vi "Set 2D Picture Ring.vi"(8 "error in (no error)":errorcluster, 10 "Selection Grid":T1) -> (0 "error out":errorcluster, 1 "Valid":bool, 3 "Grassfire out":refnum<class "Grassfire.lvclass">)   [LabVIEW 2019, in "Grassfire.lvclass"]
uses:
  Grassfire.lvclass
  Shared/Selection--array.ctl
  Shared/Selection--picture ring.ctl
  Grassfire.lvclass/Grassfire.ctl
  Node/Node.lvclass
  Address/Address.lvclass
  Shared/Shared.lvlib
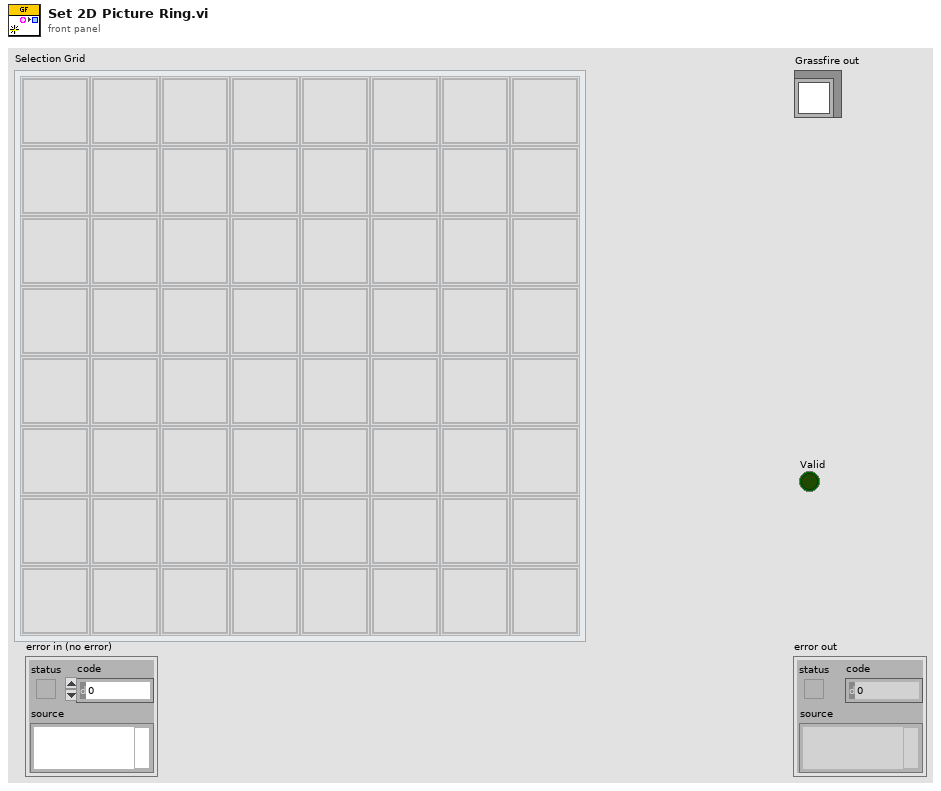
[diagram p1: front panel]
types:
  T1 = typedef "Shared.lvlib/Selection--array.ctl" = cluster{"Grid Value":T2}[][]
  T2 = typedef "Shared.lvlib/Selection--picture ring.ctl" = i64
  T3 = cluster{"Empty":refnum<class "Node.lvclass">, "Blocked":refnum<class "Node.lvclass">, "Start":refnum<class "Node.lvclass">, "End":refnum<class "Node.lvclass">, "Path":refnum<class "Node.lvclass">}
  T4 = map{refnum<class "Address.lvclass">, refnum<class "Node.lvclass">}
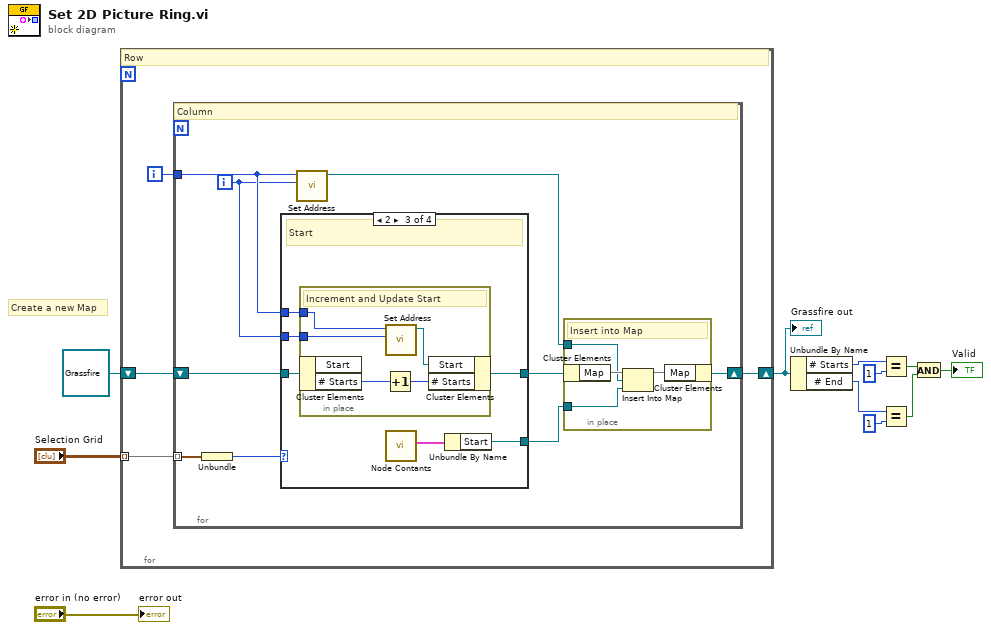
[diagram p0: block diagram]
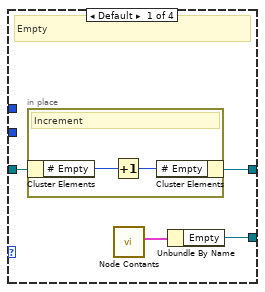
[diagram p2: hidden frame]
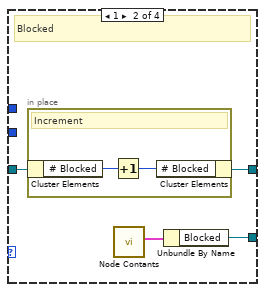
[diagram p3: hidden frame]
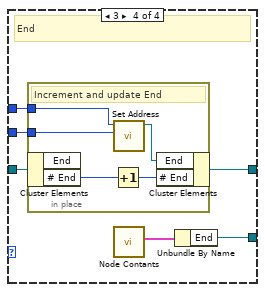
[diagram p4: hidden frame]
diagram:
  # "Create a new Map"
  n1 = for {
    tunnel: "Selection Grid" -> [w15] mode=indexing
    shift-right: [w12] -> w1
    shift-left: refnum<class "Grassfire.lvclass"> refnum ("Grassfire out") -> [w13]
    i -> [w14]
    # "Row"
    n2 = for {
      tunnel: w15 -> [w24] mode=indexing
      tunnel: w14 -> [w23]
      shift-right: [w18] -> w12
      shift-left: w13 -> [w20]
      i -> [w22]
      # "Column"
      n3 = Unbundle(w24) -> ("Grid Value"=w21:T2)
      n4 = case shown="2" w21 {
        tunnel: w20 -> [w32 w38 w46 w57]
        tunnel: [w31 w37 w45 w56] -> w19
        tunnel: w23 -> [_ _ w44 w55]
        tunnel: w22 -> [_ _ w43 w54]
        tunnel: [w29 w35 w41 w52] -> w16
        frame Default {
          # "Empty"
          n5 = in-place {
            # "Increment"
            n6 = in-place-cluster #1(w32) -> ("# Empty"=w34:i32)
            n7 = Increment(x=w34) -> (x+1=w33:i32)
            n8 = in-place-cluster #1("# Empty"=w33) -> (w31:refnum<class "Grassfire.lvclass">)
          }
          n9 = call "Node Contants.vi"() -> ("Constants"=w30:T3)  [unwired: 10 in, 1 out]
          n10 = Unbundle By Name(w30) -> ("Empty"=w29:refnum<class "Node.lvclass">)
        }
        frame 1 {
          # "Blocked"
          n11 = in-place {
            # "Increment"
            n12 = in-place-cluster #2(w38) -> ("# Blocked"=w40:i32)
            n13 = Increment(x=w40) -> (x+1=w39:i32)
            n14 = in-place-cluster #2("# Blocked"=w39) -> (w37:refnum<class "Grassfire.lvclass">)
          }
          n15 = call "Node Contants.vi"() -> ("Constants"=w36:T3)  [unwired: 10 in, 1 out]
          n16 = Unbundle By Name(w36) -> ("Blocked"=w35:refnum<class "Node.lvclass">)
        }
        frame 2 {
          # "Start"
          n17 = in-place {
            in-place-border: w44 -> [w49]
            in-place-border: w43 -> [w48]
            # "Increment and Update Start"
            n18 = in-place-cluster #3(w46) -> ("# Starts"=w51:i32)  [unwired: 1 out]
            n19 = Increment(x=w51) -> (x+1=w50:i32)
            n20 = call "Set Address.vi"("Column"=w48, "Row"=w49) -> ("2D Array Index"=w47:refnum<class "Address.lvclass">)  [unwired: 9 in]
            n21 = in-place-cluster #3("Start"=w47, "# Starts"=w50) -> (w45:refnum<class "Grassfire.lvclass">)
          }
          n22 = call "Node Contants.vi"() -> ("Constants"=w42:T3)  [unwired: 10 in, 1 out]
          n23 = Unbundle By Name(w42) -> ("Start"=w41:refnum<class "Node.lvclass">)
        }
        frame 3 {
          # "End"
          n24 = in-place {
            in-place-border: w55 -> [w60]
            in-place-border: w54 -> [w59]
            # "Increment and update End"
            n25 = in-place-cluster #4(w57) -> ("# End"=w62:i32)  [unwired: 1 out]
            n26 = Increment(x=w62) -> (x+1=w61:i32)
            n27 = call "Set Address.vi"("Column"=w59, "Row"=w60) -> ("2D Array Index"=w58:refnum<class "Address.lvclass">)  [unwired: 9 in]
            n28 = in-place-cluster #4("End"=w58, "# End"=w61) -> (w56:refnum<class "Grassfire.lvclass">)
          }
          n29 = call "Node Contants.vi"() -> ("Constants"=w53:T3)  [unwired: 10 in, 1 out]
          n30 = Unbundle By Name(w53) -> ("End"=w52:refnum<class "Node.lvclass">)
        }
      }
      n31 = call "Set Address.vi"("Column"=w22, "Row"=w23) -> ("2D Array Index"=w17:refnum<class "Address.lvclass">)  [unwired: 9 in]
      n32 = in-place {
        in-place-border: w17 -> [w26]
        in-place-border: w16 -> [w25]
        # "Insert into Map"
        n33 = in-place-cluster #5(w19) -> ("Map"=w28:T4)
        n34 = Insert Into Map(map in=w28, key=w26, value=w25) -> (map out=w27:T4)  [unwired: 2 out]
        n35 = in-place-cluster #5("Map"=w27) -> (w18:refnum<class "Grassfire.lvclass">)
      }
    }
  }
  "Grassfire out" <- w1
  n36 = Unbundle By Name(w1) -> ("# Starts"=w4:i32, "# End"=w3:i32)
  n37 = Equal?(x=w4, y=1) -> (x = y?=w7:bool)
  n38 = Equal?(x=w3, y=1) -> (x = y?=w5:bool)
  n39 = And(x=w7, y=w5) -> (x .and. y?=→"Valid":bool)
  "error out" <- "error in (no error)"
